vi "OP80_DATECODE_02_29_07_PM.vi"() -> ()   [LabVIEW 2020]
panel:
  in  "OP80_DATECODE":T1
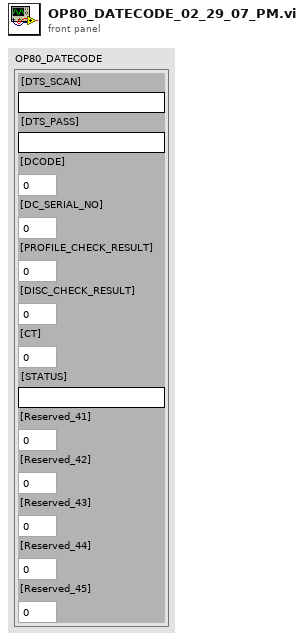
[diagram p1: front panel]
types:
  T1 = cluster{"[DTS_SCAN]":string, "[DTS_PASS]":string, "[DCODE]":dbl, "[DC_SERIAL_NO]":dbl, "[PROFILE_CHECK_RESULT]":dbl, "[DISC_CHECK_RESULT]":dbl, "[CT]":dbl, "[STATUS]":string, "[Reserved_41]":dbl, "[Reserved_42]":dbl, "[Reserved_43]":dbl, "[Reserved_44]":dbl, "[Reserved_45]":dbl}
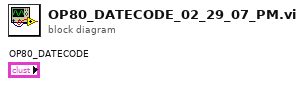
[diagram p0: block diagram]
diagram:
